vi "Hanging.vi"(8 "Climb?":bool, 10 "Hanging":cluster{"Erection MotorControlDeviceRef":T2}={"Erection MotorControlDeviceRef"={"DeviceStatus"={"status"=FALSE, "code"=0, "source"=""}, "Type"=enum."PWM", "PWM"={"PWM Channel"=enum."Invalid", "DeadBand"={"Name"="", "maxPositivePwm"=0, "minPositivePwm"=0, "centerPwm"=0, "maxNegativePwm"=0, "minNegativePwm"=0, "angularRange"=0}}, "CAN"={"Device Number"=0, "Control Mode"=enum."Percent VBus", "Semaphore"=refnum, "Max Vout"=12.0, "TalonSRX Control Mode"=enum."Percent VBus"}, "Invert"=FALSE}}, 11 "Pneumatics":T12={"CompressorDevRef"={"DevStatus"={"status"=FALSE, "code"=0, "source"=""}, "Pneumatics Control Module"=0}, "High and Low Gear DoubleSolenoidDevRef"={"DevStatus"={"status"=FALSE, "code"=0, "source"=""}, "Pneumatics Control Module"=0, "Forward Solenoid Channel"=enum."Invalid", "Reverse Solenoid Channel"=enum."Invalid"}, "PTO SingleSolenoidDevRef"={"DevStatus"={"status"=FALSE, "code"=0, "source"=""}, "Pneumatics Control Module"=0, "Forward Solenoid Channel"=enum."Invalid", "Reverse Solenoid Channel"=enum."Invalid"}, "Shooter SolenoidDevRef"={"DevStatus"={"status"=FALSE, "code"=0, "source"=""}, "Pneumatics Control Module"=0, "Forward Solenoid Channel"=enum."Invalid", "Reverse Solenoid Channel"=enum."Invalid"}, "Drive Neutral SolenoidDevRef"={"DevStatus"={"status"=FALSE, "code"=0, "source"=""}, "Pneumatics Control Module"=0, "Forward Solenoid Channel"=enum."Invalid", "Reverse Solenoid Channel"=enum."Invalid"}}) -> (2 "Hanging":cluster{"Erection MotorControlDeviceRef":T2}={"Erection MotorControlDeviceRef"={"DeviceStatus"={"status"=FALSE, "code"=0, "source"=""}, "Type"=enum."PWM", "PWM"={"PWM Channel"=enum."Invalid", "DeadBand"={"Name"="", "maxPositivePwm"=0, "minPositivePwm"=0, "centerPwm"=0, "maxNegativePwm"=0, "minNegativePwm"=0, "angularRange"=0}}, "CAN"={"Device Number"=0, "Control Mode"=enum."Percent VBus", "Semaphore"=refnum, "Max Vout"=12.0, "TalonSRX Control Mode"=enum."Percent VBus"}, "Invert"=FALSE}}, 3 "Pneumatics":T12={"CompressorDevRef"={"DevStatus"={"status"=FALSE, "code"=0, "source"=""}, "Pneumatics Control Module"=0}, "High and Low Gear DoubleSolenoidDevRef"={"DevStatus"={"status"=FALSE, "code"=0, "source"=""}, "Pneumatics Control Module"=0, "Forward Solenoid Channel"=enum."Invalid", "Reverse Solenoid Channel"=enum."Invalid"}, "PTO SingleSolenoidDevRef"={"DevStatus"={"status"=FALSE, "code"=0, "source"=""}, "Pneumatics Control Module"=0, "Forward Solenoid Channel"=enum."Invalid", "Reverse Solenoid Channel"=enum."Invalid"}, "Shooter SolenoidDevRef"={"DevStatus"={"status"=FALSE, "code"=0, "source"=""}, "Pneumatics Control Module"=0, "Forward Solenoid Channel"=enum."Invalid", "Reverse Solenoid Channel"=enum."Invalid"}, "Drive Neutral SolenoidDevRef"={"DevStatus"={"status"=FALSE, "code"=0, "source"=""}, "Pneumatics Control Module"=0, "Forward Solenoid Channel"=enum."Invalid", "Reverse Solenoid Channel"=enum."Invalid"}})   [LabVIEW 2015]
uses:
  <vilib>/Rock Robotics/WPI/Compressor/WPI_CompressorDevRef.ctl
  <vilib>/Rock Robotics/WPI/Solenoid/WPI_SolenoidDevRef.ctl
  <vilib>/Rock Robotics/WPI/Solenoid/WPI_SolenoidChannel.ctl
  <vilib>/Rock Robotics/WPI/MotorControl/WPI_MotorControlDeviceRef.ctl
  <vilib>/Rock Robotics/WPI/MotorControl/WPI_MotorControlType.ctl
  <vilib>/Rock Robotics/SystemInterfaces/DIO/FPGA_DIOPWMChannel.ctl
  <vilib>/Rock Robotics/WPI/PWM/WPI_PWMDeadband.ctl
  <vilib>/Rock Robotics/WPI/CAN/Jaguar/SubVIs/WPI_CANJaguar_ControlMode.ctl
  <vilib>/Rock Robotics/WPI/CAN/TalonSRX/WPI_CANTalonSRX_APIControlMode.ctl
  <vilib>/Rock Robotics/WPI/Solenoid/WPI_SolenoidValue.ctl
  Robot Values.vi
  <vilib>/Rock Robotics/WPI/Solenoid/WPI_SolenoidSetEnum.vi
  <vilib>/addons/control/pid/NI_PID_pid.lvlib
  <vilib>/addons/control/pid/pid.llb/PID (DBL).vi
panel:
  in  "PID gains":T1={"proportional gain (Kc)"=0.0029999999999999792, "integral time (Ti, min)"=0.01, "derivative time (Td, min)"=0.0} {"derivative time (Td, min)" format="%.3f"; "integral time (Ti, min)" format="%.3f"; "proportional gain (Kc)" format="%.3f"}
  in  "setpoint":dbl format="%.2f"
  out "Limit?":bool
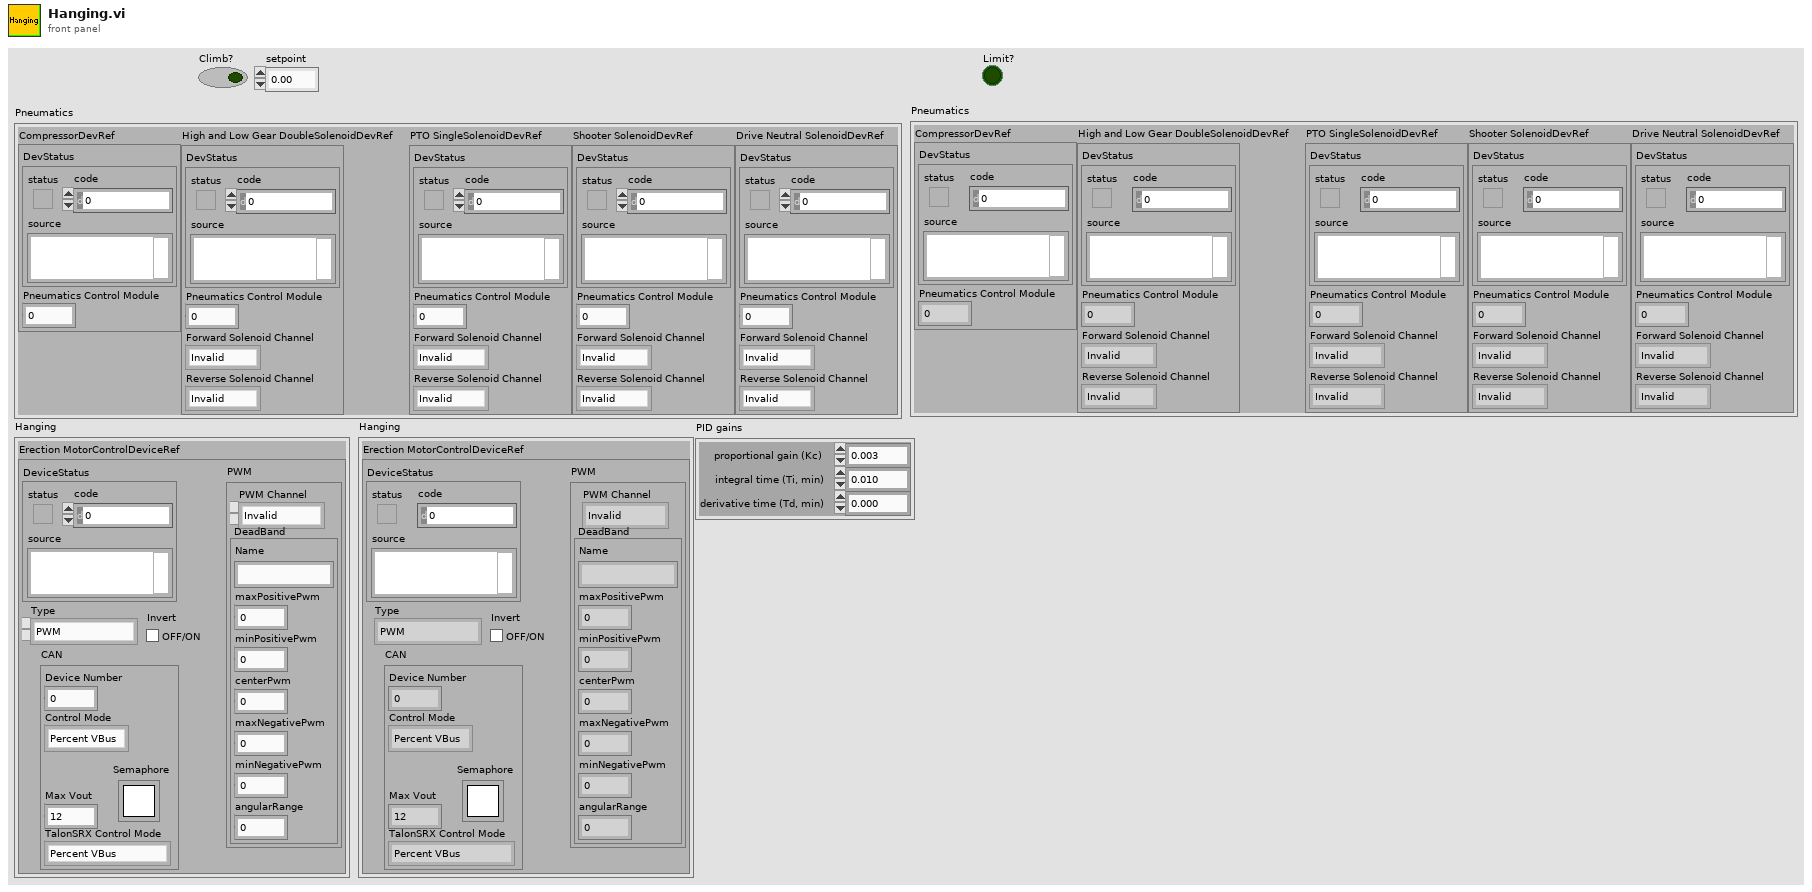
[diagram p1: front panel]
types:
  T1 = cluster{"proportional gain (Kc)":dbl, "integral time (Ti, min)":dbl, "derivative time (Td, min)":dbl}
  T2 = typedef "WPI_MotorControlDeviceRef.ctl" = cluster{"DeviceStatus":errorcluster, "Type":T3, "PWM":cluster{"PWM Channel":T4, "DeadBand":T5}, "CAN":cluster{"Device Number":u8, "Control Mode":T6, "Semaphore":T7, "Max Vout":dbl, "TalonSRX Control Mode":T8}, "Invert":bool}
  T3 = typedef "WPI_MotorControlType.ctl" = enum16{"PWM", "CAN", "CANTalonSRX"}
  T4 = typedef "FPGA_DIOPWMChannel.ctl" = enum8{"PWM 0", "PWM 1", "PWM 2", "PWM 3", "PWM 4", "PWM 5", "PWM 6", "PWM 7", "PWM 8", "PWM 9", "PWM MXP 0", "PWM MXP 1", "PWM MXP 2", "PWM MXP 3", "PWM MXP 4", "PWM MXP 5", "PWM MXP 6", "PWM MXP 7", "PWM MXP 8", "PWM MXP 9", "Invalid"}
  T5 = typedef "WPI_PWMDeadband.ctl" = cluster{"Name":string, "maxPositivePwm":i32, "minPositivePwm":i32, "centerPwm":i32, "maxNegativePwm":i32, "minNegativePwm":i32, "angularRange":u16}
  T6 = typedef "WPI_CANJaguar_ControlMode.ctl" = enum8{"Percent VBus", "Current", "Speed", "Position", "Voltage"}
  T7 = typedef "Semaphore RefNum" = refnum<k1>
  T8 = typedef "WPI_CANTalonSRX_APIControlMode.ctl" = enum8{"Percent VBus", "Speed", "Position", "Slave", "Unchanged / Invalid", "Voltage Compensation", "Current", "Motion Profile"}
  T9 = typedef "WPI_CompressorDevRef.ctl" = cluster{"DevStatus":errorcluster, "Pneumatics Control Module":u8}
  T10 = typedef "WPI_SolenoidDevRef.ctl" = cluster{"DevStatus":errorcluster, "Pneumatics Control Module":u8, "Forward Solenoid Channel":T11, "Reverse Solenoid Channel":T11}
  T11 = typedef "WPI_SolenoidChannel.ctl" = enum8{"Solenoid 0", "Solenoid 1", "Solenoid 2", "Solenoid 3", "Solenoid 4", "Solenoid 5", "Solenoid 6", "Solenoid 7", "Invalid"}
  T12 = cluster{"CompressorDevRef":T9, "High and Low Gear DoubleSolenoidDevRef":T10, "PTO SingleSolenoidDevRef":T10, "Shooter SolenoidDevRef":T10, "Drive Neutral SolenoidDevRef":T10}
  T13 = typedef "Drive Values.ctl" = cluster{"Drive Motors":cluster{"Left Motor Value":dbl, "Right Motor Value":dbl, "Left Motor Encoder":dbl, "Right Motor Encoder":dbl}, "Sensors":cluster{"Gyro Angle":dbl, "Hanging Limit":bool, "Photoeye":bool, "Ultrasonic Range":dbl, "Shooter Speed Encoder":dbl}, "Arms":cluster{"Arm Position":dbl, "Left Arm Encoder":dbl, "Right Arm Encoder":dbl, "Left Arm Lower Limit":bool, "Right Arm Lower Limit":bool}, "Acquisition and Scoring":cluster{"Acquiring?":bool}}
  T14 = typedef "WPI_SolenoidValue.ctl" = enum16{"Off", "On", "Forward", "Reverse"}
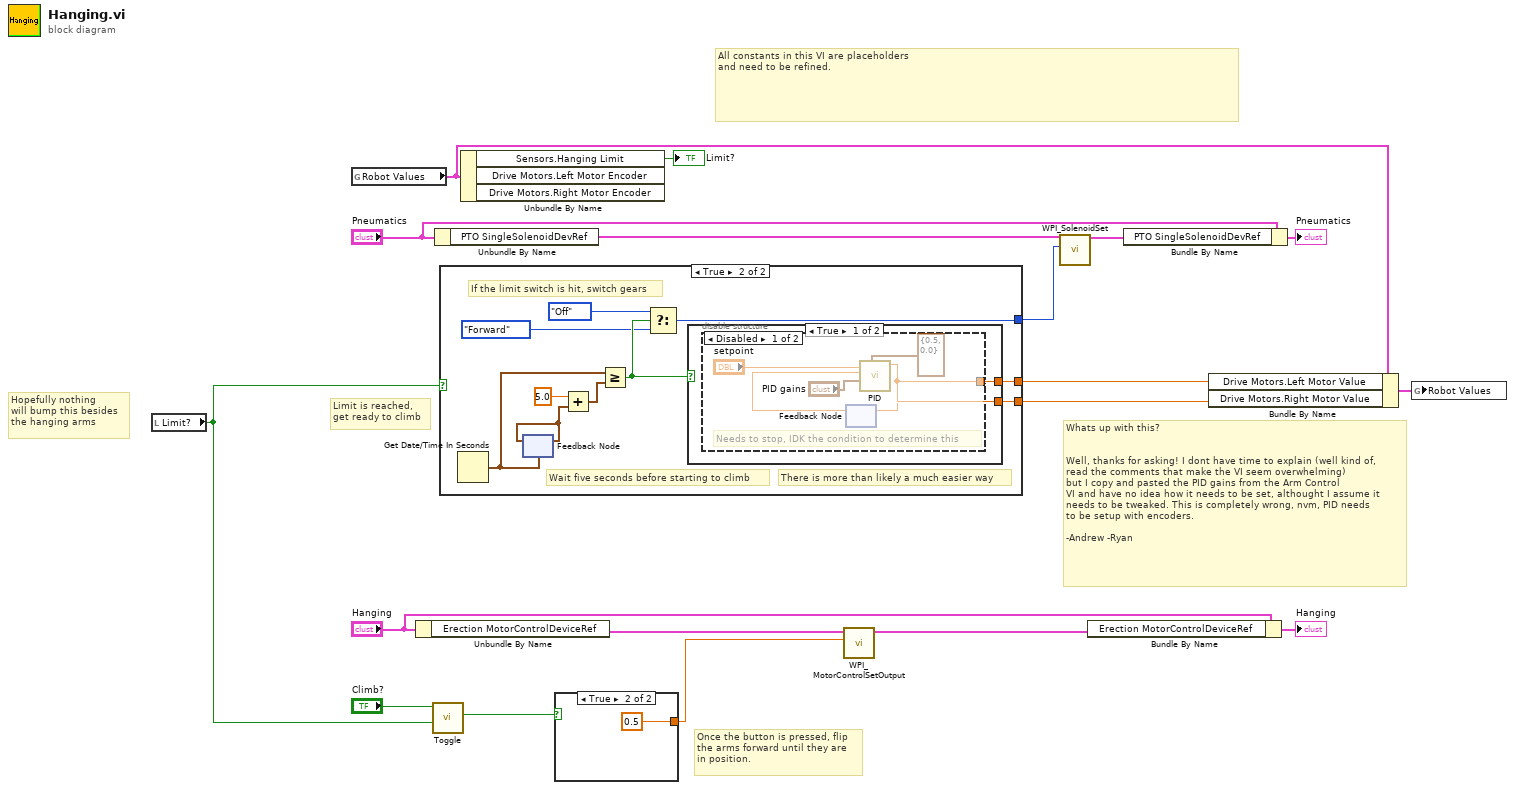
[diagram p0: block diagram]
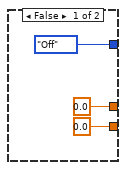
[diagram p2: hidden frame]
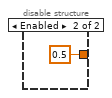
[diagram p3: hidden frame]
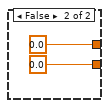
[diagram p4: hidden frame]
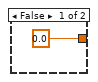
[diagram p5: hidden frame]
diagram:
  # "Whats up with this?\n\n\nWell, thanks for asking! I dont have time to explain (well kind of, \nread the comments that make the VI seem overwhelming)\nbut I copy and pasted the PID gains from the Arm Control\nVI and have no idea how it needs to be set, althought I assume it\nneeds to be tweaked. This is completely wrong, nvm, PID needs\nto be setup with encoders.\n\n-Andrew -Ryan"
  # "Hopefully nothing\nwill bump this besides\nthe hanging arms"
  # "Limit is reached,\nget ready to climb"
  # "All constants in this VI are placeholders\nand need to be refined."
  # "Once the button is pressed, flip\nthe arms forward until they are\nin position."
  n1 = local read "Limit?"() -> (w4:bool)
  n2 = global read "Robot Values.vi" "Robot Values"() -> (w17:T13)
  n3 = Unbundle By Name("Hanging") -> ("Erection MotorControlDeviceRef"=w11:T2)
  n4 = call "Toggle.vi"("Internal Toggle"=w4, "User Toggle"="Climb?") -> ("True/False"=w7:bool)  [unwired: 9 in]
  n5 = Unbundle By Name("Pneumatics") -> ("PTO SingleSolenoidDevRef"=w10:T10)
  n6 = case shown="True" w4 {
    tunnel: [WPI_SolenoidValue."Off" ("Value") w27] -> w3
    tunnel: [0.0 w26] -> w2
    tunnel: [0.0 w25] -> w1
    frame False {
    }
    frame True {
      # "If the limit switch is hit, switch gears"
      # "Wait five seconds before starting to climb"
      # "There is more than likely a much easier way"
      n7 = Get Date/Time In Seconds() -> (seconds since 1Jan1904=w28:timestamp)
      n8 = feedback #1(w28) -> (w30:timestamp)
      n9 = feedback-in #1(w30) -> ()
      n10 = Add(x=5.0, y=w30) -> (x+y=w31:timestamp)
      n11 = Greater Or Equal?(x=w28, y=w31) -> (x >= y?=w24:bool)
      n12 = Select(t=WPI_SolenoidValue."Off" ("f"), s=w24, f=WPI_SolenoidValue."Forward" ("Value")) -> (s? t:f=w27:T14)
      n13 = case shown="True" w24 {
        tunnel: [w32 0.0] -> w26
        tunnel: [w32 0.0] -> w25
        frame True {
          n14 = disable-structure shown="Disabled" {
            disable-tunnel: [w37 0.5 ("output")] -> w32
            frame Disabled {
              # "Needs to stop, IDK the condition to determine this"
              n15 = feedback #2() -> (w36:dbl)  [unwired: 1 in]
              n16 = call-poly <vilib>:"PID.vi"("output range"=cluster{"output high":dbl, "output low":dbl} {"output high"=0.5, "output low"=0.0}, "PID gains"="PID gains", "process variable"=w36, "setpoint"="setpoint") -> ("output"=w37:dbl)  [unwired: 6 in, 1 out]
              n17 = feedback-in #2(w37) -> ()
            }
            frame Enabled {
            }
          }
        }
        frame False {
        }
      }
    }
  }
  n18 = Unbundle By Name(w17) -> ("Sensors.Hanging Limit"=→"Limit?":bool)  [unwired: 2 out]
  n19 = case shown="True" w7 {
    tunnel: [0.0 0.5] -> w8
    frame False {
    }
    frame True {
    }
  }
  n20 = call <vilib>:"WPI_MotorControlSetOutput.vi"("Output"=w8, "MotorControlDevRef"=w11) -> ("MotorControlDevRef"=w12:T2)  [unwired: 7 in, 2 out]
  n21 = call-poly <vilib>:"WPI_SolenoidSet.vi"("Value"=w3, "SolenoidDevRef"=w10) -> ("SolenoidDevRef"=w9:T10)  [unwired: 8 in, 1 out]
  n22 = Bundle By Name(cluster="Hanging", "Erection MotorControlDeviceRef"=w12) -> (→"Hanging":cluster{"Erection MotorControlDeviceRef":T2})
  n23 = Bundle By Name(cluster="Pneumatics", "PTO SingleSolenoidDevRef"=w9) -> (→"Pneumatics":T12)
  n24 = Bundle By Name(cluster=w17, "Drive Motors.Left Motor Value"=w2, "Drive Motors.Right Motor Value"=w1) -> (w18:T13)
  n25 = global write "Robot Values.vi" "Robot Values"(w18) -> ()
